vi "Installed Classes to Rings.vi"(8 "error in (no error)":errorcluster, 9 "Installed":refnum<class "Instrument.lvclass">[](array[class]), 10 "Rings":refnum<vi>[](array[refnum]), 11 "C.E.":refnum<class "Control Experiment.lvclass">) -> (0 "error out":errorcluster, 3 "C.E. out":refnum<class "Control Experiment.lvclass">)   [LabVIEW 2019, in "Control Experiment.lvclass"]
uses:
  Control Experiment.lvclass
  <userlib>/LevyLab/Instrument Framework/Instrument/Instrument.lvclass
  Typedefs/Instrument Types--enum.ctl
  Control Experiment.lvclass/Control Experiment.ctl
  C:/Program Files/National Instruments/LabVIEW 2019/vi.lib/JKI/JKI SMO/SMO/SMO.lvclass
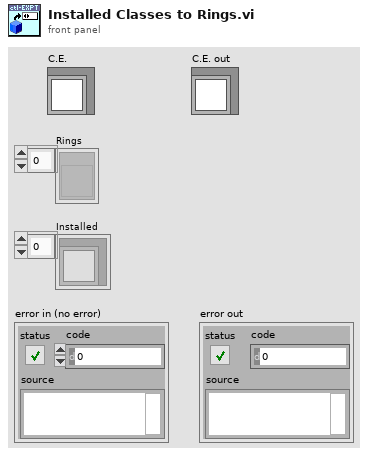
[diagram p1: front panel]
types:
  T1 = typedef "Control Experiment.lvclass/Instrument Types--enum.ctl" = enum16{"DAQ", "Amplifier", "Temperature", "Magnet", "Rotator", "Level", "Capacitance", "Delay Line", "Strain Cell", "VNA", "Source"}
  T2 = typedef "Control Experiment.lvclass/Instruments--cluster.ctl" = cluster{"class path":path, "Address":string, "Type":T1}
  T3 = typedef "LVStringsAndValuesArrayTypeDef.ctl" = cluster{"String":string, "Value":ext}[]
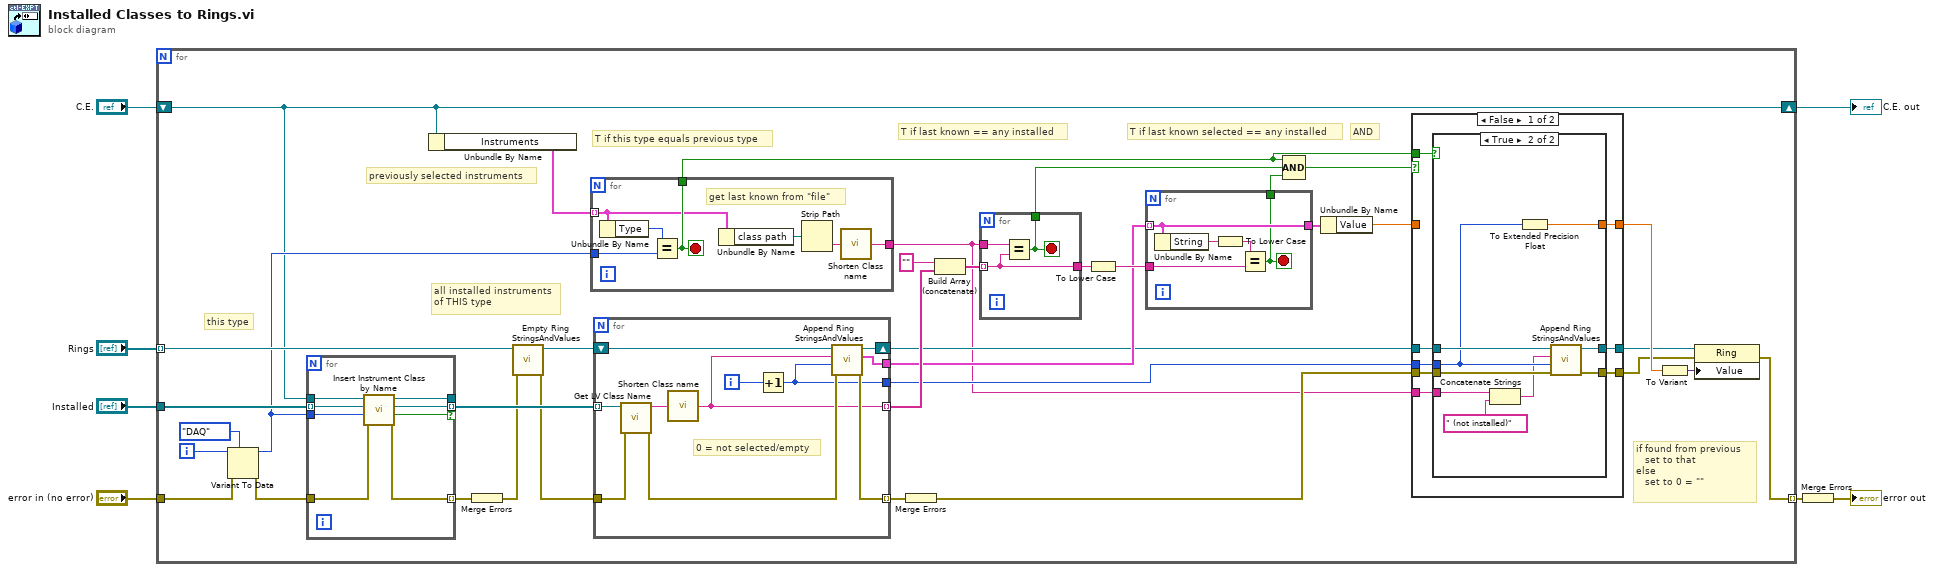
[diagram p0: block diagram]
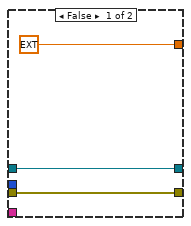
[diagram p2: hidden frame]
diagram:
  n1 = for {
    tunnel: "Rings" -> [w43] mode=indexing
    tunnel: "Installed" -> [w42]
    shift-right: [w18] -> w1
    shift-left: "C.E." -> [w18]
    tunnel: "error in (no error)" -> [w41]
    tunnel: [w40] -> w4 mode=indexing
    i -> [w39]
    # "all installed instruments\nof THIS type"
    # "previously selected instruments"
    # "if found from previous\n   set to that\nelse\n   set to 0 = \"\""
    # "AND"
    # "T if last known selected == any installed"
    # "T if this type equals previous type"
    # "T if last known == any installed"
    # "this type"
    n2 = Variant To Data(error in=w41, type=Instrument_Types--enum."DAQ" ("Type"), Variant=w39) -> (data=w21:T1, error out=w20:errorcluster)
    n3 = for {
      tunnel: w42 -> [w70] mode=indexing
      tunnel: [w73] -> w29 mode=indexing if=w67
      tunnel: w20 -> [w74]
      tunnel: w18 -> [w72]
      tunnel: [w71] -> _
      tunnel: [w69] -> w28 mode=indexing
      tunnel: w21 -> [w68]
      n4 = call "Insert Instrument Class by Name.vi"("error in (no error)"=w74, "Type"=w68, "Instrument in"=w70, "Control Experiment in"=w72) -> ("error out"=w69:errorcluster, "Found?"=w67:bool, "Instrument out"=w73:refnum<class "Instrument.lvclass">, "Control Experiment out"=w71:refnum<class "Control Experiment.lvclass">)  [unwired: 4 in]
    }
    n5 = Unbundle By Name(w18) -> ("Instruments"=w36:T2[])
    n6 = Merge Errors(w28) -> (w24:errorcluster)
    n7 = call "Empty Ring StringsAndValues.vi"("error in (no error)"=w24, "Ring in"=w43) -> ("error out"=w25:errorcluster, "Ring out"=w30:refnum<vi>)  [unwired: 8 in]
    n8 = for {
      tunnel: w36 -> [w77] mode=indexing
      tunnel: w21 -> [w80]
      tunnel: [w79] -> w14
      tunnel: [w75] -> w8
      stop <- w79 stop-if-true
      # "get last known from \"file\""
      n9 = Unbundle By Name(w77) -> ("Type"=w81:T1)
      n10 = Equal?(x=w81, y=w80) -> (x = y?=w79:bool)
      n11 = Unbundle By Name(w77) -> ("class path"=w78:path)
      n12 = Strip Path(path=w78) -> (name=w76:string)  [unwired: 1 out]
      n13 = call "Shorten Class name.vi"("Qualified Class Name"=w76) -> ("Name"=w75:string)
    }
    n14 = for {
      tunnel: [w84] -> w37 mode=indexing
      tunnel: w29 -> [w92] mode=indexing
      tunnel: [w88] -> w19
      tunnel: w25 -> [w86]
      tunnel: [w83] -> w23 mode=indexing
      shift-right: [w89] -> w13
      shift-left: w30 -> [w91]
      tunnel: [w82] -> w11
      i -> [w90]
      # "0 = not selected/empty"
      n15 = call <vilib>:"Get LV Class Name.vi"("error in (no error)"=w86, "object"=w92) -> ("error out"=w85:errorcluster, "class name"=w87:string)  [unwired: 8 in]
      n16 = call "Shorten Class name.vi"("Qualified Class Name"=w87) -> ("Name"=w83:string)
      n17 = Increment(x=w90) -> (x+1=w82:i32)
      n18 = call "Append Ring StringsAndValues.vi"("error in (no error)"=w85, "Value"=w82, "String"=w83, "Ring in"=w91) -> ("error out"=w84:errorcluster, "StringsAndValues[]"=w88:T3, "Ring out"=w89:refnum<vi>)  [unwired: 5 in]
    }
    n19 = Merge Errors(w37) -> (w10:errorcluster)
    n20 = Build Array (concatenate)("", w23) -> (w32:string[])
    n21 = for {
      tunnel: w32 -> [w93] mode=indexing
      tunnel: w8 -> [w94]
      tunnel: [w93] -> w27
      tunnel: [w95] -> w34
      stop <- w95 stop-if-true
      n22 = Equal?(x=w94, y=w93) -> (x = y?=w95:bool)
    }
    n23 = To Lower Case(string=w27) -> (all lower case string=w31:string)
    n24 = for {
      tunnel: w19 -> [w98] mode=indexing
      tunnel: w31 -> [w99]
      tunnel: [w98] -> w38
      tunnel: [w97] -> w35
      stop <- w97 stop-if-true
      n25 = Unbundle By Name(w98) -> ("String"=w100:string)
      n26 = To Lower Case(string=w100) -> (all lower case string=w96:string)
      n27 = Equal?(x=w96, y=w99) -> (x = y?=w97:bool)
    }
    n28 = Compound Arithmetic op=AND(w14, w34, w35) -> (w17:bool)
    n29 = Unbundle By Name(w38) -> ("Value"=w16:ext)
    n30 = case shown="False" w17 {
      tunnel: w16 -> [_ w66]
      tunnel: [w50 w66] -> w15
      tunnel: w14 -> [w51 _]
      tunnel: w13 -> [w49 w65]
      tunnel: [w48 w65] -> w12
      tunnel: w11 -> [w47 _]
      tunnel: w10 -> [w46 w64]
      tunnel: [w45 w64] -> w9
      tunnel: w8 -> [w44 _]
      frame False {
        n31 = case shown="True" w51 {
          tunnel: [ext 0.0 ("Value") w61] -> w50
          tunnel: w49 -> [w52 w63]
          tunnel: [w52 w62] -> w48
          tunnel: w47 -> [_ w58]
          tunnel: w46 -> [w53 w60]
          tunnel: [w53 w59] -> w45
          tunnel: w44 -> [_ w55]
          frame False {
          }
          frame True {
            n32 = Concatenate Strings(w55, " (not installed)" ("format string")) -> (w56:string)
            n33 = To Extended Precision Float(1:w58) -> (0:w61:ext)
            n34 = call "Append Ring StringsAndValues.vi"("error in (no error)"=w60, "Value"=w58, "String"=w56, "Ring in"=w63) -> ("error out"=w59:errorcluster, "Ring out"=w62:refnum<vi>)  [unwired: 5 in, 1 out]
          }
        }
      }
      frame True {
      }
    }
    n35 = To Variant(anything=w15) -> (Variant=w26:variant)
    n36 = property class="Ring"(reference=w12, error in=w9, "Value"=w26) -> (error out=w40:errorcluster)  [unwired: 1 out]
  }
  "C.E. out" <- w1
  n37 = Merge Errors(w4) -> (→"error out":errorcluster)
